vi "line_density.vi"(1 "DensCurr":dbl[](array[numeric])) -> (0 "Line Density":dbl)   [LabVIEW 2015]
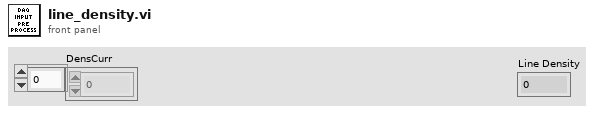
[diagram p1: front panel]
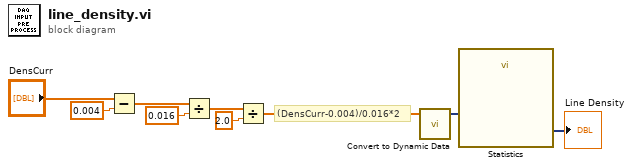
[diagram p0: block diagram]
diagram:
  # "(DensCurr-0.004)/0.016*2"
  n1 = Subtract(x="DensCurr", y=0.004) -> (x-y=w8:dbl[])
  n2 = Divide(x=w8, y=0.016) -> (x/y=w6:dbl[])
  n3 = Divide(x=w6, y=2.0) -> (x/y=w3:dbl[])
  n4 = call "Convert to Dynamic Data"("Array"=w3) -> ("Dynamic Data Type"=w2:dynamicdata)  [unwired: 3 in]
  n5 = call "Statistics"("Signals"=w2) -> ("Arithmetic Mean"=→"Line Density":dynamicdata)  [unwired: 25 in, 1 out]
